vi "HTTP.Header String to Dictionary.vi"(10 "HTTP Header":string) -> (2 "Dictionary":variant)   [LabVIEW 2013, in "Connection.WS_GOSPL.lvlib" / "Connection.WS.lvclass"]
uses:
  Connection.WS.lvclass
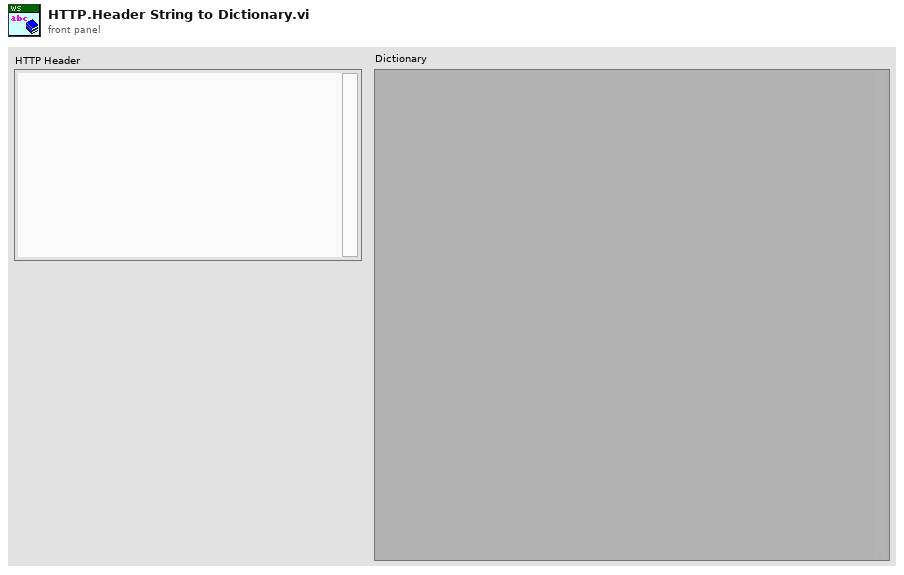
[diagram p1: front panel]
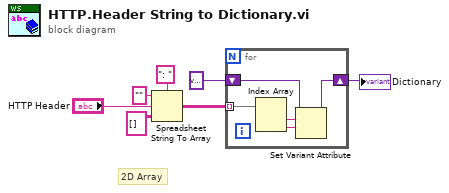
[diagram p0: block diagram]
diagram:
  # "2D Array"
  n1 = Spreadsheet String To Array(delimiter (Tab)=": ", format string="", spreadsheet string="HTTP Header", array type (2D Dbl)=string[][] []) -> (array=w2:string[][])
  n2 = for {
    shift-right: [w8] -> w3
    shift-left: variant ("variant") -> [w12]
    tunnel: w2 -> [w11] mode=indexing
    n3 = Index Array(array=w11) -> (element #1=w10:string, element #2=w9:string)  [unwired: 2 in]
    n4 = Set Variant Attribute(Variant=w12, name=w10, value=w9) -> (Variant out=w8:variant)  [unwired: 1 in, 2 out]
  }
  "Dictionary" <- w3
